vi "Head Nod Example.vi"   [LabVIEW 2016]
doc: "Example VI: Nods Baxter's head twice"
panel:
  # "Hit run to nod the head"
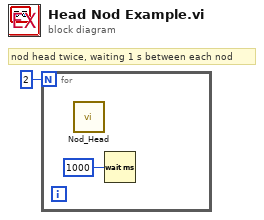
[diagram p0: block diagram]
diagram:
  # "nod head twice, waiting 1 s between each nod"
  n1 = for {
    N: 2 -> [_]
    n2 = call "Nod_Head.vi"() -> ()  [unwired: 4 in, 1 out]
    n3 = Wait (ms)(milliseconds to wait=u32 1000) -> ()  [unwired: 1 out]
  }
